vi "invalid_connection.vi"(8 "error in (no error)":errorcluster, 11 "TCP Connection in":refnum<class "TCP Connection.lvclass">) -> (0 "error out":errorcluster, 1 "invalid connection?":bool, 3 "TCP Connection out":refnum<class "TCP Connection.lvclass">)   [LabVIEW 2019, in "TCP Connection.lvclass"]
uses:
  TCP Connection.lvclass
  TCP Connection.lvclass/TCP Connection.ctl
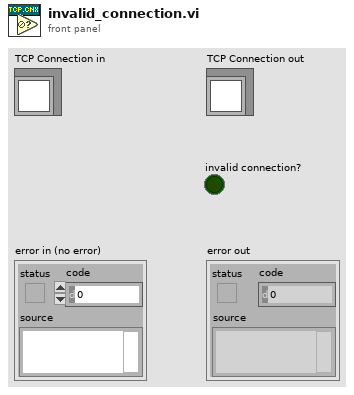
[diagram p1: front panel]
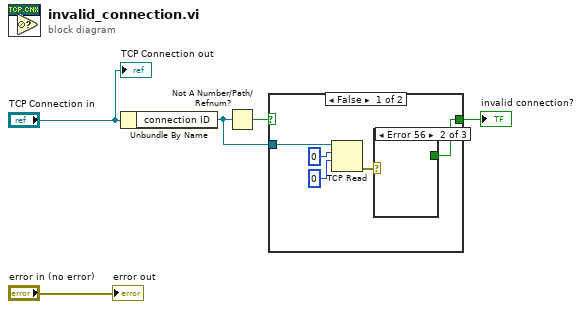
[diagram p0: block diagram]
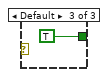
[diagram p3: hidden frame]
diagram:
  n1 = Unbundle By Name("TCP Connection in") -> ("connection ID"=w3:refnum<k5>)
  n2 = Not A Number/Path/Refnum?(number/path/refnum=w3) -> (NaN/Path/Refnum?=w2:bool)
  n3 = case shown="False" w2 {
    selector: w2 -> [_ w12]
    tunnel: w3 -> [w10 _]
    tunnel: [w6 w12] -> w1
    frame False {
      n4 = TCP Read(connection ID=w10, bytes to read=0, 9:0 ("timeout ms (25000)")) -> (error out=w7:errorcluster)  [unwired: 2 in, 2 out]
      n5 = case shown="Error 56" w7 {
        tunnel: [_ _ TRUE] -> w6
        frame No Error {
        }
        frame Error {
        }
        frame Default {
        }
      }
    }
    frame True {
    }
  }
  "invalid connection?" <- w1
  "error out" <- "error in (no error)"
  "TCP Connection out" <- "TCP Connection in"
